vi "BuildTileCode32.vi"(4 "replacecolor 2":fxp<+,3,3>, 5 "replacecolor":fxp<+,3,3>, 6 "color_to_replace 2":fxp<+,3,3>, 7 "color_to_replace":fxp<+,3,3>, 9 "Flip":enum16{"None", "LeftRight", "UpDown", "Both"}(ring), 10 "Rotation":enum16{"None", "Right", "Down", "Left"}(ring), 11 "Tilenumber":u16) -> (3 "TileCode":u32)   [LabVIEW 2019, in "RT_Game.lvlib" / "Engine.lvclass"]
uses:
  Engine.lvclass
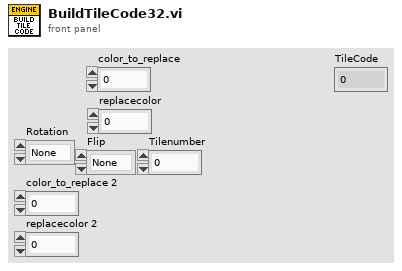
[diagram p1: front panel]
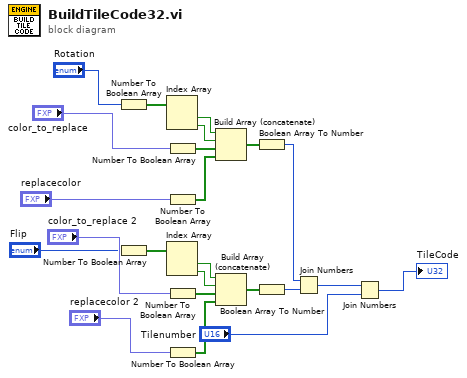
[diagram p0: block diagram]
diagram:
  n1 = Number To Boolean Array(number="Rotation") -> (Boolean array=w14:bool[])
  n2 = Number To Boolean Array(number="Flip") -> (Boolean array=w6:bool[])
  n3 = Index Array(array=w14) -> (element #1=w13:bool, element #2=w12:bool)  [unwired: 2 in]
  n4 = Index Array(array=w6) -> (element #1=w7:bool, element #2=w8:bool)  [unwired: 2 in]
  n5 = Number To Boolean Array(number="color_to_replace") -> (Boolean array=w11:bool[])
  n6 = Number To Boolean Array(number="replacecolor") -> (Boolean array=w15:bool[])
  n7 = Number To Boolean Array(number="color_to_replace 2") -> (Boolean array=w9:bool[])
  n8 = Number To Boolean Array(number="replacecolor 2") -> (Boolean array=w16:bool[])
  n9 = Build Array (concatenate)(w13, w12, w11, w15) -> (w10:bool[])
  n10 = Build Array (concatenate)(w7, w8, w9, w16) -> (w5:bool[])
  n11 = Boolean Array To Number(Boolean array=w10) -> (number=w3:u8)
  n12 = Boolean Array To Number(Boolean array=w5) -> (number=w2:u8)
  n13 = Join Numbers(hi=w3, lo=w2) -> ((hi.lo)=w4:u16)
  n14 = Join Numbers(hi=w4, lo="Tilenumber") -> ((hi.lo)=→"TileCode":u32)
